vi "Plot_data_fr_file_mod.vi"() -> ()   [LabVIEW 2010]
uses:
  Anemometry/Anemometry Sub Vis/Controls/In_Range.ctl
panel:
  out "Plot 3":cluster{dbl[], dbl[]}[](graph)
  out "Plot 2":cluster{dbl[], dbl[]}[](graph)
  in  "Today":bool
  out "Second taken":dbl=0.316 format="%.2f"
  in  "Data folder location":string="G3_3 HD:EnFlo data:"
  in  "End Date":T1={"day of month"=9, "month"=10, "year"=2000} {"year" min=1998 max=2100}
  in  "Start Date":T1={"day of month"=9, "month"=10, "year"=2000} {"year" min=1998 max=2100}
  in  "Selector 1":i32[](listbox)
  out "Plot":cluster{dbl[], dbl[]}[](graph)
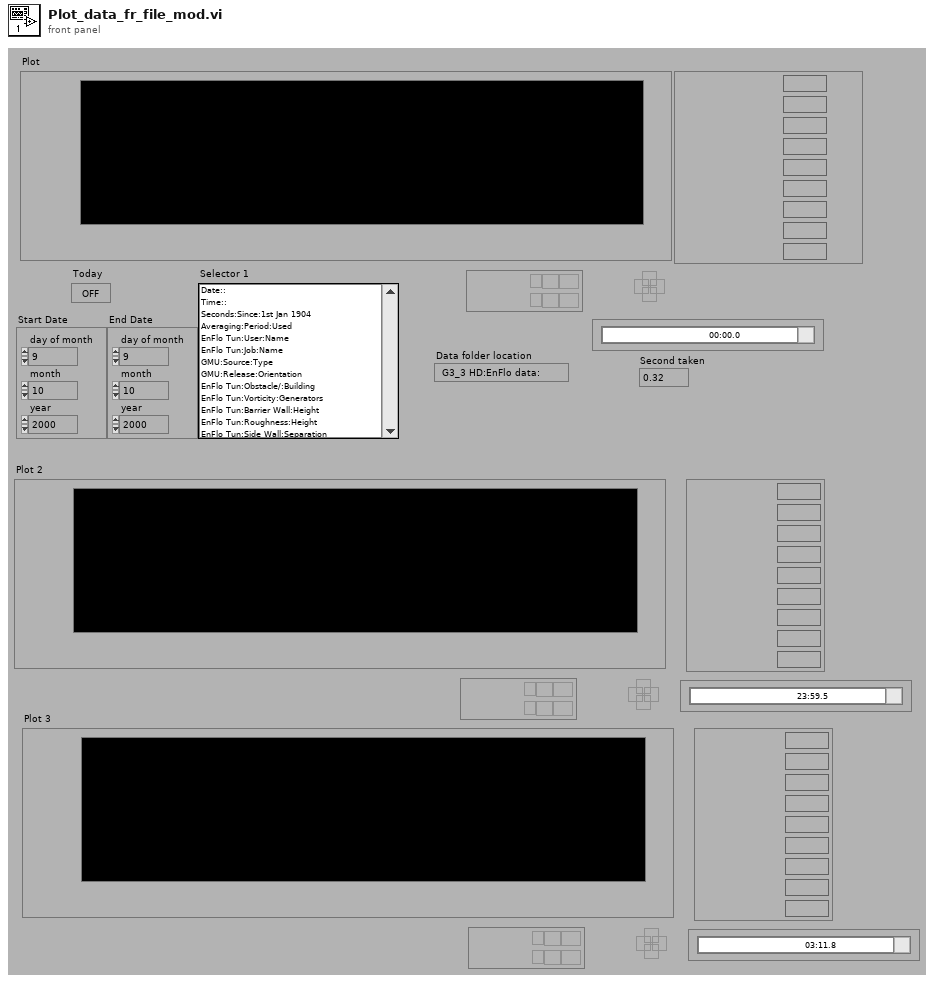
[diagram p1: front panel]
types:
  T1 = cluster{"day of month":i32, "month":i32, "year":i32}
  T2 = cluster{"second":i32, "minute":i32, "hour":i32, "day of month":i32, "month":i32, "year":i32, "day of week":i32, "day of year":i32, "is DST":i32}
  T3 = typedef "In_Range.ctl" = enum16{"%", "±", "% & ±"}
  T4 = cluster{"day of month":i32, "month":i32, "year":i32}[]
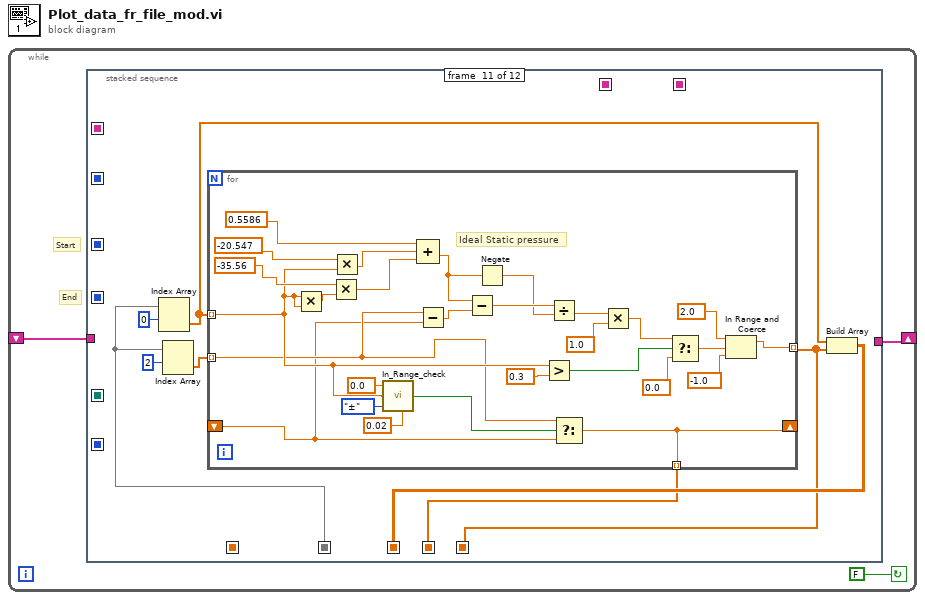
[diagram p0: block diagram]
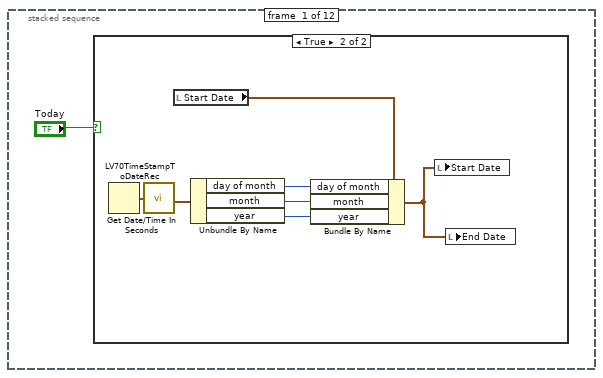
[diagram p2: hidden frame]
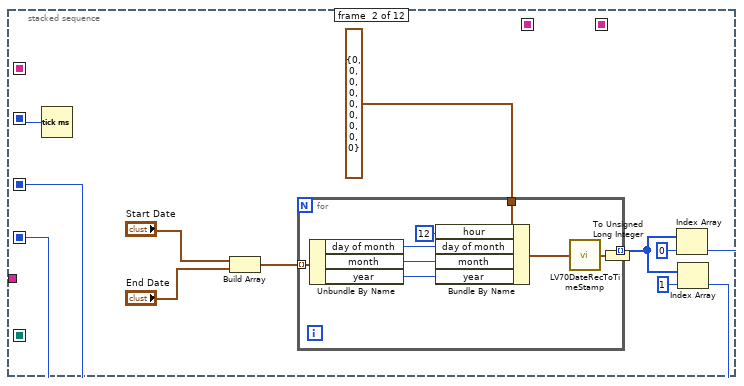
[diagram p4: hidden frame]
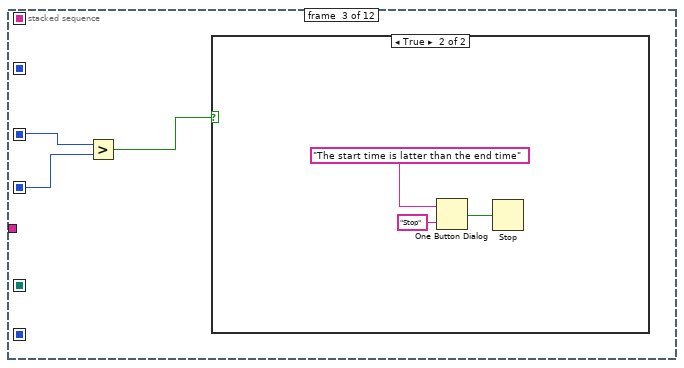
[diagram p5: hidden frame]
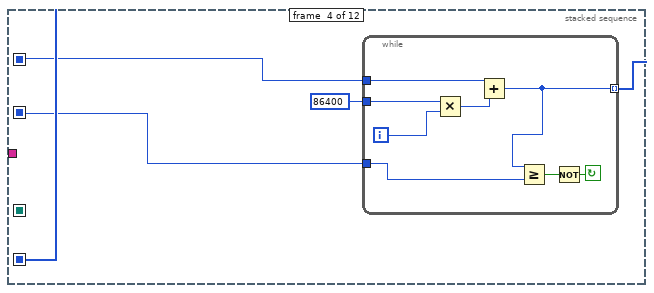
[diagram p7: hidden frame]
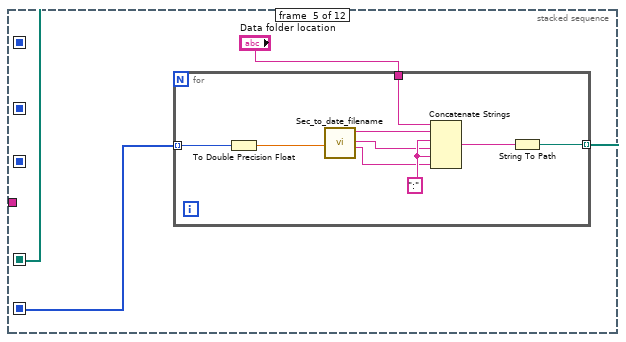
[diagram p8: hidden frame]
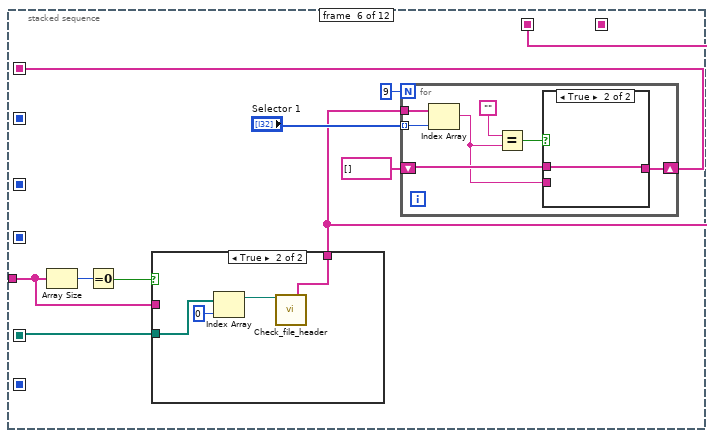
[diagram p9: hidden frame]
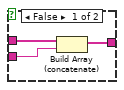
[diagram p11: hidden frame]
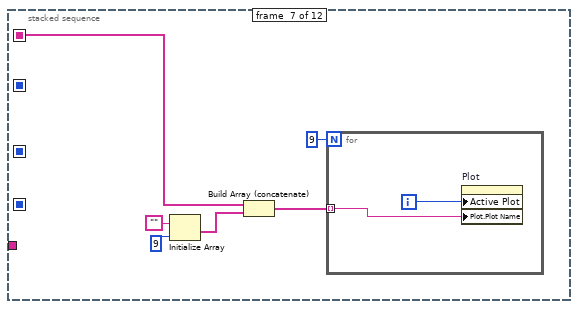
[diagram p12: hidden frame]
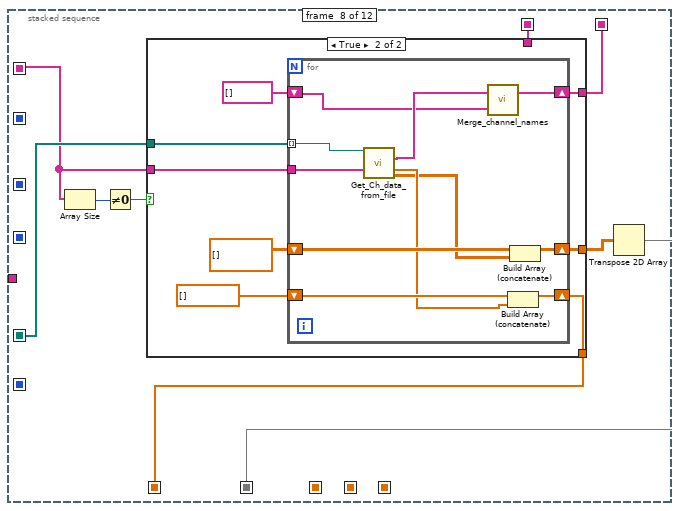
[diagram p13: hidden frame]
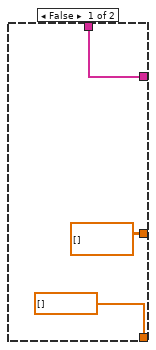
[diagram p14: hidden frame]
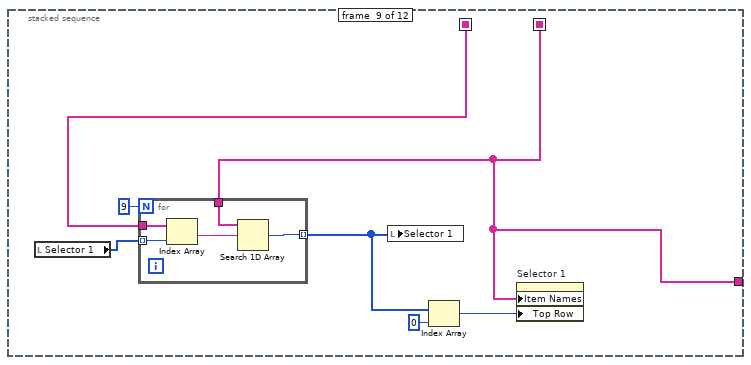
[diagram p15: hidden frame]
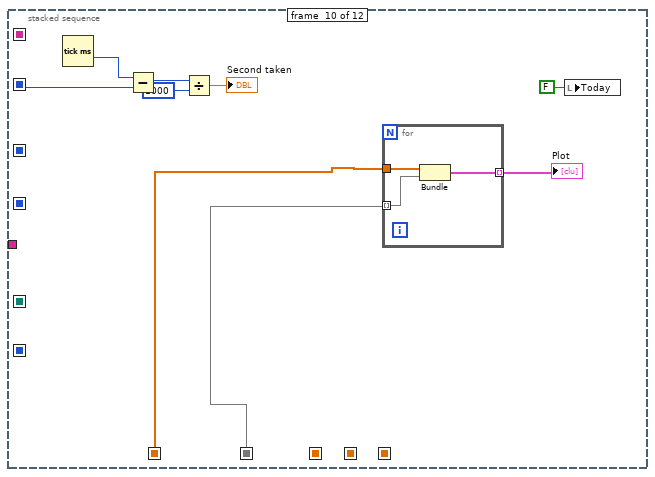
[diagram p16: hidden frame]
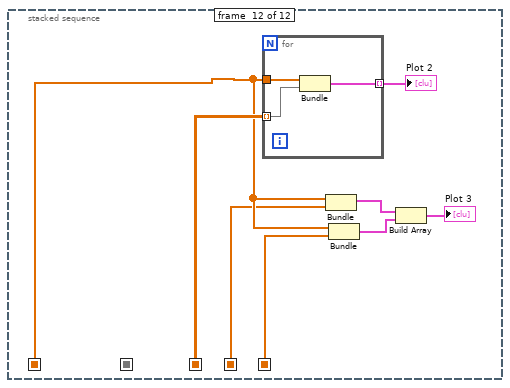
[diagram p17: hidden frame]
diagram:
  n1 = while {
    shift-left: _ -> [w2]
    shift-right: [w3] -> _
    stop <- FALSE continue-if-true
    # "End"
    # "Start"
    n2 = stacked-sequence {
      seq-local: [_ _ _ w40 _ _ _ _ _ _ _ _] -> [_ _ _ _ w51 _ _ _ _ _ _ _]
      seq-local: [_ _ _ _ w50 _ _ _ _ _ _ _] -> [_ _ _ _ _ w69 _ w102 _ _ _ _]
      seq-local: [_ _ _ _ _ w61 _ _ _ _ _ _] -> [_ _ _ _ _ _ w89 w97 _ _ _ _]
      seq-local: [_ _ _ _ _ _ _ w101 _ _ _ _] -> [_ _ _ _ _ _ _ _ _ w143 _ w190]
      seq-local: [_ _ _ _ _ _ _ w99 _ _ _ _] -> [_ _ _ _ _ _ _ _ _ w145 w154 _]
      seq-local: [_ w16 _ _ _ _ _ _ _ _ _ _] -> [_ _ w32 w39 _ _ _ _ _ _ _ _]
      seq-local: [_ w15 _ _ _ _ _ _ _ _ _ _] -> [_ _ w33 w38 _ _ _ _ _ _ _ _]
      seq-local: [_ _ _ _ _ _ _ w98 _ _ _ _] -> [_ _ _ _ _ _ _ _ w126 _ _ _]
      seq-local: [_ _ _ _ _ w64 _ _ _ _ _ _] -> [_ _ _ _ _ _ _ w94 w129 _ _ _]
      seq-local: [_ w13 _ _ _ _ _ _ _ _ _ _] -> [_ _ _ _ _ _ _ _ _ w141 _ _]
      seq-local: [_ _ _ _ _ _ _ _ _ _ w151 _] -> [_ _ _ _ _ _ _ _ _ _ _ w191]
      seq-local: [_ _ _ _ _ _ _ _ _ _ w150 _] -> [_ _ _ _ _ _ _ _ _ _ _ w189]
      seq-local: [_ _ _ _ _ _ _ _ _ _ w149 _] -> [_ _ _ _ _ _ _ _ _ _ _ w185]
      tunnel: [_ _ _ _ _ _ _ _ w126 _ _ _] -> w3
      tunnel: w2 -> [_ _ _ _ _ w65 _ _ _ _ _ _]
      frame #0 {
        n3 = case shown="True" "Today" {
          frame False {
          }
          frame True {
            n4 = Get Date/Time In Seconds() -> (seconds since 1Jan1904=w5:timestamp)
            n5 = call <vilib>:"LV70TimeStampToDateRec.vi"("time stamp"=w5) -> ("date time rec"=w11:T2)
            n6 = local read "Start Date"() -> (w10:T1)
            n7 = Unbundle By Name(w11) -> ("day of month"=w9:i32, "month"=w8:i32, "year"=w7:i32)
            n8 = Bundle By Name(cluster=w10, "day of month"=w9, "month"=w8, "year"=w7) -> (w6:T1)
            n9 = local write "Start Date"(w6) -> ()
            n10 = local write "End Date"(w6) -> ()
          }
        }
      }
      frame #1 {
        n11 = Tick Count (ms)() -> (millisecond timer value=w13:u32)
        n12 = Build Array("Start Date", "End Date") -> (w19:T4)
        n13 = for {
          tunnel: T2 {"second"=0, "minute"=0, "hour"=0, "day of month"=0, "month"=0, "year"=0, "day of week"=0, "day of year"=0, "is DST"=0} ("date time rec") -> [w30]
          tunnel: w19 -> [w24] mode=indexing
          tunnel: [w23] -> w14 mode=indexing
          n14 = Unbundle By Name(w24) -> ("day of month"=w29:i32, "month"=w28:i32, "year"=w27:i32)
          n15 = Bundle By Name(cluster=w30, "hour"=12, "day of month"=w29, "month"=w28, "year"=w27) -> (w25:T2)
          n16 = call <vilib>:"LV70DateRecToTimeStamp.vi"("date time rec"=w25) -> ("Time Stamp"=w22:timestamp)
          n17 = To Unsigned Long Integer(number=w22) -> (unsigned 32bit integer=w23:u32)
        }
        n18 = Index Array(array=w14, index=0) -> (element=w16:u32)
        n19 = Index Array(array=w14, index=1) -> (element=w15:u32)
      }
      frame #2 {
        n20 = Greater?(x=w32, y=w33) -> (0:w31:bool)
        n21 = case shown="True" w31 {
          frame False {
          }
          frame True {
            n22 = One Button Dialog(message="The start time is latter than the end time", button name ("OK")="Stop") -> (true=w35:bool)
            n23 = Stop(stop? (T)=w35) -> ()
          }
        }
      }
      frame #3 {
        n24 = while {
          tunnel: [w41] -> w40 mode=indexing
          tunnel: w38 -> [w48]
          tunnel: w39 -> [w42]
          tunnel: u32 86400 ("seconds") -> [w44]
          i -> [w45]
          stop <- w46 continue-if-true
          n25 = Multiply(x=w44, y=w45) -> (x*y=w43:u32)
          n26 = Add(x=w42, y=w43) -> (x+y=w41:u32)
          n27 = Greater Or Equal?(x=w41, y=w48) -> (x >= y?=w47:bool)
          n28 = Not(x=w47) -> (.not. x?=w46:bool)
        }
      }
      frame #4 {
        n29 = for {
          tunnel: w51 -> [w56] mode=indexing
          tunnel: "Data folder location" -> [w54]
          tunnel: [w52] -> w50 mode=indexing
          w60 = ":"
          n30 = To Double Precision Float(number=w56) -> (double precision float=w55:dbl)
          n31 = call "Sec_to_date_filename.vi"("seconds"=w55) -> ("Year"=w57:string, "Month"=w58:string, "Day"=w59:string)  [unwired: 1 out]
          n32 = Concatenate Strings(w54, w57, w60, w58, w60, w59) -> (w53:string)
          n33 = String To Path(string=w53) -> (path=w52:path)
        }
      }
      frame #5 {
        n34 = Array Size(array=w65) -> (size(s)=w67:i32)
        n35 = Equal To 0?(x=w67) -> (x = 0?=w66:bool)
        n36 = case shown="True" w66 {
          tunnel: w69 -> [_ w73]
          tunnel: [w70 w71] -> w64
          tunnel: w65 -> [w70 _]
          frame False {
          }
          frame True {
            n37 = Index Array(array=w73, index=0) -> (element=w72:path)
            n38 = call "Check_file_header.vi"("Filename"=w72) -> ("File Channels"=w71:string[])  [unwired: 3 in, 11 out]
          }
        }
        n39 = for {
          N: 9 -> [_]
          tunnel: "Selector 1" -> [w81] mode=indexing
          tunnel: w64 -> [w80]
          shift-right: [w76] -> w61
          shift-left: string[] [] -> [w77]
          n40 = Index Array(array=w80, index=w81) -> (element=w75:string)
          n41 = Equal?(x="", y=w75) -> (x = y?=w78:bool)
          n42 = case shown="True" w78 {
            tunnel: w77 -> [w84 w85]
            tunnel: [w83 w85] -> w76
            tunnel: w75 -> [w82 _]
            frame False {
              n43 = Build Array (concatenate)(w84, w82) -> (w83:string[])
            }
            frame True {
            }
          }
        }
      }
      frame #6 {
        n44 = Initialize Array("", 9) -> (w88:string[])
        n45 = Build Array (concatenate)(w89, w88) -> (w87:string[])
        n46 = for {
          N: 9 -> [_]
          tunnel: w87 -> [w92] mode=indexing
          i -> [w93]
          n47 = property on="Plot" class="XYGraph (strict)"("Active Plot"=w93, "Plot.Plot Name"=w92) -> ()  [unwired: 2 in, 2 out]
        }
      }
      frame #7 {
        n48 = Array Size(array=w97) -> (size(s)=w96:i32)
        n49 = Not Equal To 0?(x=w96) -> (x != 0?=w95:bool)
        n50 = case shown="True" w95 {
          tunnel: w102 -> [_ w113]
          tunnel: [dbl[] [] w110] -> w101
          tunnel: [dbl[][] [] w109] -> w100
          tunnel: [w103 w107] -> w98
          tunnel: w97 -> [_ w106]
          tunnel: w94 -> [w103 _]
          frame False {
          }
          frame True {
            n51 = for {
              tunnel: w113 -> [w124] mode=indexing
              shift-right: [w122] -> w109
              shift-left: dbl[][] [] -> [w123]
              shift-right: [w121] -> w110
              shift-left: dbl[] [] -> [w120]
              shift-right: [w115] -> w107
              shift-left: string[] [] ("Merged Channels") -> [w116]
              tunnel: w106 -> [w114]
              n52 = call "Get_Ch_data_from_file.vi"("Filename"=w124, "Channel names"=w114) -> ("File Channels"=w117:string[], "Times"=w119:dbl[], "Ch Data"=w118:dbl[][])  [unwired: 2 in, 9 out]
              n53 = call "Merge_channel_names.vi"("Preferred Channel array"=w117, "Channel array"=w116) -> ("Merged Channels"=w115:string[])  [unwired: 2 out]
              n54 = Build Array (concatenate)(w120, w119) -> (w121:dbl[])
              n55 = Build Array (concatenate)(w123, w118) -> (w122:dbl[][])
            }
          }
        }
        n56 = Transpose 2D Array(2D array=w100) -> (transposed array=w99:dbl[][])
      }
      frame #8 {
        n57 = local read "Selector 1"() -> (w130:i32[])
        n58 = for {
          N: 9 -> [_]
          tunnel: w130 -> [w136] mode=indexing
          tunnel: [w135] -> w127 mode=indexing
          tunnel: w129 -> [w134]
          tunnel: w126 -> [w132]
          n59 = Index Array(array=w134, index=w136) -> (element=w133:string)
          n60 = Search 1D Array(1D array=w132, element=w133) -> (index of element=w135:i32)  [unwired: 1 out]
        }
        n61 = local write "Selector 1"(w127) -> ()
        n62 = Index Array(array=w127, index=0) -> (element=w128:i32)
        n63 = property on="Selector 1" class="LstBox (strict)"("Item Names"=w126, "Top Row"=w128) -> ()  [unwired: 2 in, 2 out]
      }
      frame #9 {
        n64 = Tick Count (ms)() -> (millisecond timer value=w142:u32)
        n65 = Subtract(x=w142, y=w141) -> (x-y=w140:u32)
        n66 = Divide(x=w140, y=u32 1000) -> (x/y=→"Second taken":dbl)
        n67 = for {
          tunnel: w143 -> [w148]
          tunnel: w145 -> [w147] mode=indexing
          tunnel: [w146] -> w144 mode=indexing
          n68 = Bundle(w148, w147) -> (w146:cluster{dbl[], dbl[]})  [unwired: 1 out]
        }
        "Plot" <- w144
        n69 = local write "Today"(FALSE ("Today")) -> ()
      }
      frame #10 {
        n70 = Index Array(array=w154, index (row)=0 ("Index")) -> (element=w152:dbl[])  [unwired: 1 in]
        n71 = Index Array(array=w154, index (row)=2 ("Index")) -> (element=w153:dbl[])  [unwired: 1 in]
        n72 = for {
          tunnel: w153 -> [w161] mode=indexing
          tunnel: w152 -> [w166] mode=indexing
          tunnel: [w157] -> w150 mode=indexing
          shift-right: [w158] -> _
          shift-left: _ -> [w160]
          tunnel: [w158] -> w149 mode=indexing
          # "Ideal Static pressure"
          n73 = Multiply(x=w166, y=w166) -> (x*y=w183:dbl)
          n74 = Multiply(x=-35.56, y=w183) -> (x*y=w182:dbl)
          n75 = Multiply(x=-20.547, y=w166) -> (x*y=w184:dbl)
          n76 = call "In_Range_check.vi"("±"=0.02, "Mode"=In_Range."±", "Value"=w166, "Setpoint"=0.0) -> ("In Range"=w162:bool)  [unwired: 1 in, 2 out]
          n77 = Compound Arithmetic op=ADD(0.5586, w184, w182) -> (w180:dbl)
          n78 = Subtract(x=w161, y=w160) -> (x-y=w159:dbl)
          n79 = Subtract(x=w180, y=w159) -> (x-y=w181:dbl)
          n80 = Negate(x=w180) -> (-x=w179:dbl)
          n81 = Greater?(x=w166, y=0.3) -> (0:w175:bool)
          n82 = Divide(x=w181, y=w179) -> (x/y=w178:dbl)
          n83 = Select(t=w161, s=w162, f=w160) -> (s? t:f=w158:dbl)
          n84 = Multiply(x=w178, y=1.0) -> (x*y=w174:dbl)
          n85 = Select(t=w174, s=w175, f=0.0) -> (s? t:f=w173:dbl)
          n86 = In Range and Coerce(upper limit=2.0 ("Max"), x=w173, lower limit=-1.0 ("Min")) -> (coerced(x)=w157:dbl)  [unwired: 1 out]
        }
        n87 = Build Array(w152, w150) -> (w151:dbl[][])
      }
      frame #11 {
        n88 = for {
          tunnel: w190 -> [w195]
          tunnel: w191 -> [w194] mode=indexing
          tunnel: [w193] -> w192 mode=indexing
          n89 = Bundle(w195, w194) -> (w193:cluster{dbl[], dbl[]})  [unwired: 1 out]
        }
        "Plot 2" <- w192
        n90 = Bundle(w190, w185) -> (w188:cluster{dbl[], dbl[]})  [unwired: 1 out]
        n91 = Bundle(w190, w189) -> (w187:cluster{dbl[], dbl[]})  [unwired: 1 out]
        n92 = Build Array(w188, w187) -> (→"Plot 3":cluster{dbl[], dbl[]}[])
      }
    }
  }
